vi "WriteSignal Export Cluster.vi"(8 "Error In":errorcluster, 10 "Signal Export Cluster":T1={"Export Signal"=FALSE, "Output Terminal (do not export)"="PFI0", "Signal to Export"=106} {"Signal to Export" items=["Sample Clock"=101, "Sample Clock Timebase"=1006, "Reference Clock"=102, "Onboard Reference Clock"=1019, "Start Trigger"=1004, "Script Trigger"=103, "Marker Event"=1001, "Data Marker Event"=108, "Ready For Start Event"=105, "Started Event"=106, "Done Event"=107, "Synchronization Pulse"=1007, "Sync Out"=1002]}, 11 "object in":refnum<class "Pulsetrain Config.lvclass">) -> (0 "Error Out":errorcluster, 3 "object out":refnum<class "Pulsetrain Config.lvclass">)   [LabVIEW 2023, in "Teledyne-T3AFG120.lvlib" / "Pulsetrain Config.lvclass"]
uses:
  Pulsetrain Config.lvclass
  PXI-5441_class/configurations/DC Config_class/Signal Export Cluster.ctl
  <instrlib>/niFgen/niFgen.llb/niFgen_ctl Exported Signal Desination Values (ComboBox).ctl
  <instrlib>/niFgen/niFgen.llb/niFgen_ctl Exported Signal Name Values (Ring).ctl
  Pulsetrain Config.lvclass/Pulsetrain Config.ctl
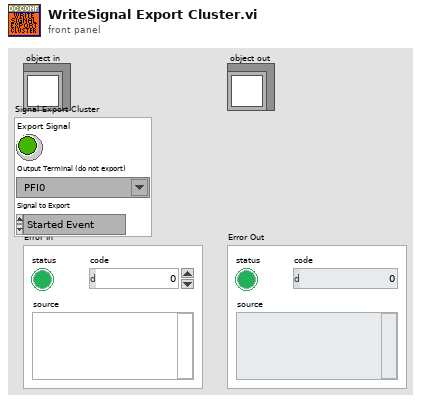
[diagram p1: front panel]
types:
  T1 = typedef "Signal Export Cluster.ctl" = cluster{"Export Signal":bool, "Output Terminal (do not export)":T2, "Signal to Export":T3}
  T2 = typedef "niFgen_ctl Exported Signal Desination Values (ComboBox).ctl" = string
  T3 = typedef "niFgen_ctl Exported Signal Name Values (Ring).ctl" = u16
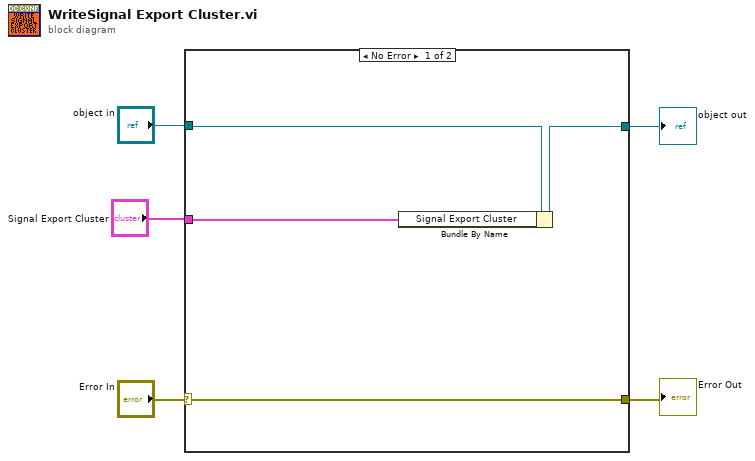
[diagram p0: block diagram]
diagram:
  n1 = case shown="No Error" "Error In" {
    selector: "Error In" -> [w8 w11]
    tunnel: [w8 w11] -> w4
    tunnel: [w6 w10] -> w2
    tunnel: "object in" -> [w7 w10]
    tunnel: "Signal Export Cluster" -> [w9 _]
    frame No Error {
      n2 = Bundle By Name(cluster=w7, "Signal Export Cluster"=w9) -> (w6:refnum<class "Pulsetrain Config.lvclass">)
    }
    frame Error {
    }
  }
  "Error Out" <- w4
  "object out" <- w2
